vi "To XML.vi"(8 "error in (no error)":errorcluster, 11 "TOC in":refnum<class "TOC.lvclass">) -> (0 "error out":errorcluster, 2 "XML String":string, 3 "TOC out":refnum<class "TOC.lvclass">)   [LabVIEW 2015, in "TOC.lvclass"]
uses:
  TOC.lvclass
  TOC.lvclass/TOC.ctl
  Topic/Topic.lvclass
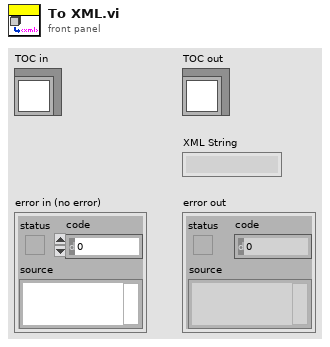
[diagram p1: front panel]
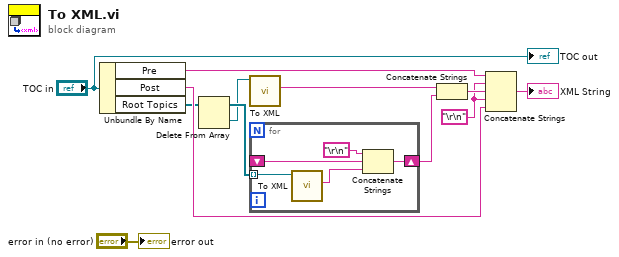
[diagram p0: block diagram]
diagram:
  w1 = "\r\n"
  n1 = Unbundle By Name("TOC in") -> ("Pre"=w10:string, "Post"=w9:string, "Root Topics"=w7:refnum<class "Topic.lvclass">[])
  n2 = Delete From Array(array=w7) -> (deleted portion=w5:refnum<class "Topic.lvclass">, array with subset deleted=w6:refnum<class "Topic.lvclass">[])  [unwired: 2 in]
  n3 = call-dynamic "To XML.vi"("Topic in"=w5) -> ("XML String"=w4:string)  [unwired: 8 in, 2 out]
  n4 = for {
    tunnel: w6 -> [w17] mode=indexing
    shift-right: [w14] -> w3
    shift-left: _ -> [w15]
    n5 = call-dynamic "To XML.vi"("Topic in"=w17) -> ("XML String"=w16:string)  [unwired: 8 in, 2 out]
    n6 = Concatenate Strings("\r\n", w15, w16) -> (w14:string)
  }
  n7 = Concatenate Strings(w4, w3) -> (w2:string)
  n8 = Concatenate Strings(w10, w1, w2, w1, w9) -> (→"XML String":string)
  "error out" <- "error in (no error)"
  "TOC out" <- "TOC in"
